vi "labview_nanonis.vi"() -> ()   [LabVIEW 2019]
uses:
  <userlib>/Nanonis Prog Interface/Nanonis Prog Interface.lvlib
panel:
  in  "stop":bool
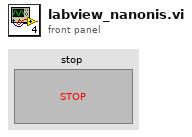
[diagram p1: front panel]
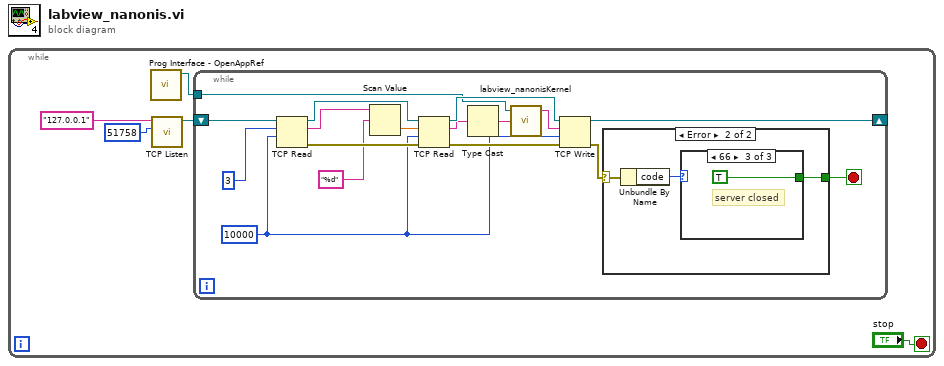
[diagram p0: block diagram]
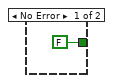
[diagram p2: hidden frame]
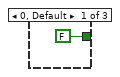
[diagram p3: hidden frame]
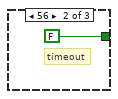
[diagram p4: hidden frame]
diagram:
  n1 = while {
    stop <- "stop" stop-if-true
    n2 = call <userlib>:"Prog Interface - OpenAppRef.vi"() -> ("Application reference"=w2:refnum<vi>)  [unwired: 6 in, 1 out]
    n3 = call <vilib>:"TCP Listen.vi"("port"=u16 51758, "service name"="127.0.0.1") -> ("connection ID"=w1:refnum<k5>)  [unwired: 5 in, 4 out]
    n4 = while {
      tunnel: w2 -> [w8]
      shift-right: [w20] -> _
      shift-left: w1 -> [w19]
      stop <- w22 stop-if-true
      w6 = 10000 ("timeout ms (25000)")
      n5 = TCP Read(connection ID=w19, bytes to read=3, 9:w6) -> (connection ID out=w17:refnum<k5>, data out=w12:string, error out=w14:errorcluster)  [unwired: 2 in]
      n6 = Scan Value(string=w12, format string="%d") -> (value=w11:dbl)  [unwired: 1 in, 1 out]
      n7 = TCP Read(connection ID=w17, bytes to read=w11, error in (no error)=w14, 9:w6) -> (connection ID out=w16:refnum<k5>, data out=w13:string, error out=w15:errorcluster)  [unwired: 1 in]
      n8 = Type Cast(x=w13) -> (*(type *) &x=w9:string)  [unwired: 1 in]
      n9 = call "labview_nanonisKernel.vi"("Input"=w9, "Application ref in"=w8) -> ("Output"=w7:string)  [unwired: 1 in, 2 out]
      n10 = TCP Write(connection ID=w16, data in=w7, error in (no error)=w15, 9:w6) -> (connection ID out=w20:refnum<k5>, error out=w21:errorcluster)  [unwired: 1 out]
      n11 = case shown="Error" w21 {
        selector: w21 -> [_ w26]
        tunnel: [FALSE w24] -> w22
        frame No Error {
        }
        frame Error {
          n12 = Unbundle By Name(w26) -> ("code"=w25:i32)
          n13 = case shown="66" w25 {
            tunnel: [FALSE FALSE TRUE] -> w24
            frame 0, Default {
            }
            frame 56 {
              # "timeout"
            }
            frame 66 {
              # "server closed"
            }
          }
        }
      }
    }
  }
